vi "test_next_steps_class.vi"(8 "error in (no error)":errorcluster) -> (0 "error out":errorcluster)   [LabVIEW 2023, in "Easy.SequenceManager.Test.lvlib"]
uses:
  Easy.SequenceManager.Test.lvlib
  src/SequenceManager/SequenceManager.lvclass
  src/Step/Step.lvclass
  <vilib>/addons/_JKI Toolkits/Caraya/classes/Assert/Assert Equal Value and Type_Variant.vi
  <vilib>/addons/_JKI Toolkits/Caraya/classes/Test/Test.lvclass
  <vilib>/addons/_JKI Toolkits/Caraya/classes/Assert/Assert.lvclass
  src/Parameter/Parameter.lvclass
panel:
  in  "SequenceManager in":refnum<class "SequenceManager.lvclass">
  # "Connector Pane"
  # "Locals"
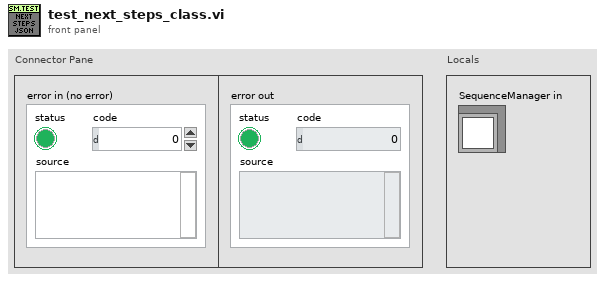
[diagram p1: front panel]
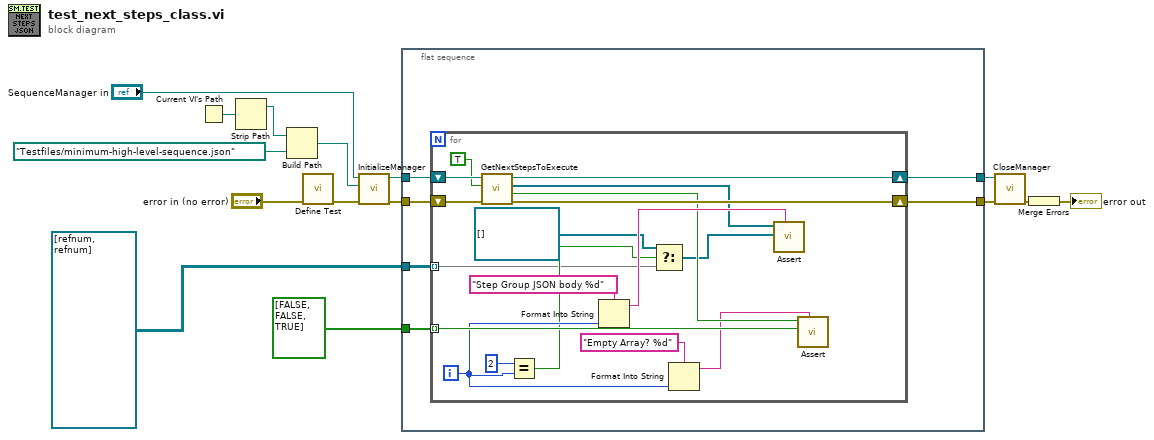
[diagram p0: block diagram]
diagram:
  n1 = Current VI's Path() -> (path=w14:path)
  n2 = Strip Path(path=w14) -> (stripped path=w8:path)  [unwired: 1 out]
  n3 = Build Path(base path=w8, name or relative path=path "Testfiles/minimum-high-level-sequence.json") -> (appended path=w9:path)
  n4 = call <vilib>:"Define Test.vi"("error in (no error)"="error in (no error)") -> ("error out"=w7:errorcluster)  [unwired: 9 in, 1 out]
  n5 = call-dynamic "InitializeManager.vi"("error in (no error)"=w7, "Path to JSON sequence file"=w9, "SequenceManager in"="SequenceManager in") -> ("error out"=w6:errorcluster, "SequenceManager out"=w10:refnum<class "SequenceManager.lvclass">)  [unwired: 7 in]
  n6 = flat-sequence {
    tunnel: w10 -> [w20]
    tunnel: w6 -> [w21]
    tunnel: [w19] -> w4
    tunnel: [w18] -> w3
    tunnel: refnum<class "Step.lvclass">[][] [[refnum], [refnum]] ("Steps") -> [w17]
    tunnel: bool[] [FALSE, FALSE, TRUE] ("Array") -> [w16]
    frame #0 {
      n7 = for {
        tunnel: w17 -> [w24] mode=indexing
        shift-right: [w36] -> w18
        shift-left: w21 -> [w39]
        shift-right: [w37] -> w19
        shift-left: w20 -> [w38]
        tunnel: w16 -> [w31] mode=indexing
        i -> [w27]
        n8 = call-dynamic "GetNextStepsToExecute.vi"("error in (no error)"=w39, "beautify JSON?"=TRUE, "SequenceManager in"=w38) -> ("error out"=w36:errorcluster, "Empty Array?"=w30:bool, "Steps"=w28:refnum<class "Step.lvclass">[], "SequenceManager out"=w37:refnum<class "SequenceManager.lvclass">)  [unwired: 5 in]
        n9 = Equal?(x=2, y=w27) -> (x = y?=w25:bool)
        n10 = Format Into String(format string="Step Group JSON body %d", w27) -> (resulting string=w33:string)  [unwired: 2 in, 1 out]
        n11 = Select(t=refnum<class "Step.lvclass">[] [] ("Steps"), s=w25, f=w24) -> (s? t:f=w22:refnum<class "Step.lvclass">[])
        n12 = Format Into String(format string="Empty Array? %d", w27) -> (resulting string=w29:string)  [unwired: 2 in, 1 out]
        n13 = call-poly <vilib>:"Assert.vi"("Label"=w33, "Y"=w22, "X"=w28) -> ()  [unwired: 7 in, 2 out]
        n14 = call-poly <vilib>:"Assert.vi"("Label"=w29, "Y"=w31, "X"=w30) -> ()  [unwired: 7 in, 2 out]
      }
    }
  }
  n15 = call-dynamic "CloseManager.vi"("error in (no error)"=w3, "SequenceManager in"=w4) -> ("error out"=w5:errorcluster)  [unwired: 8 in, 1 out]
  n16 = Merge Errors(w5) -> (→"error out":errorcluster)
